vi "Write and Convert Waveform to File.vi"(0 "File Refnum":refnum<file>, 1 "Current Supplied Voltage":dbl, 2 "Calibration State":enum16{"Idle", "Delay", "Voltage", "Response"}(ring), 5 "Waveform":waveform(dbl)[](array[waveform]), 7 "Prev Array":dbl[][](array[numeric]), 11 "error in":errorcluster) -> (4 "File Refnum Out":refnum<file>, 6 "Bridge OP Out":dbl, 10 "Shunt Volt Out":dbl, 14 "Bridge & Volt array":dbl[][](array[numeric]), 15 "error out":errorcluster)   [LabVIEW 2021]
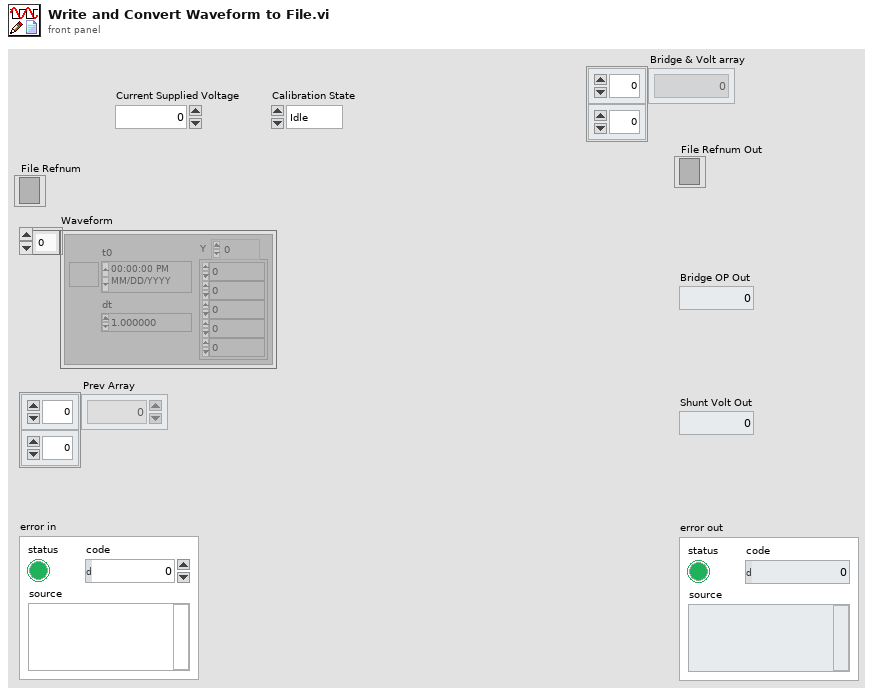
[diagram p1: front panel]
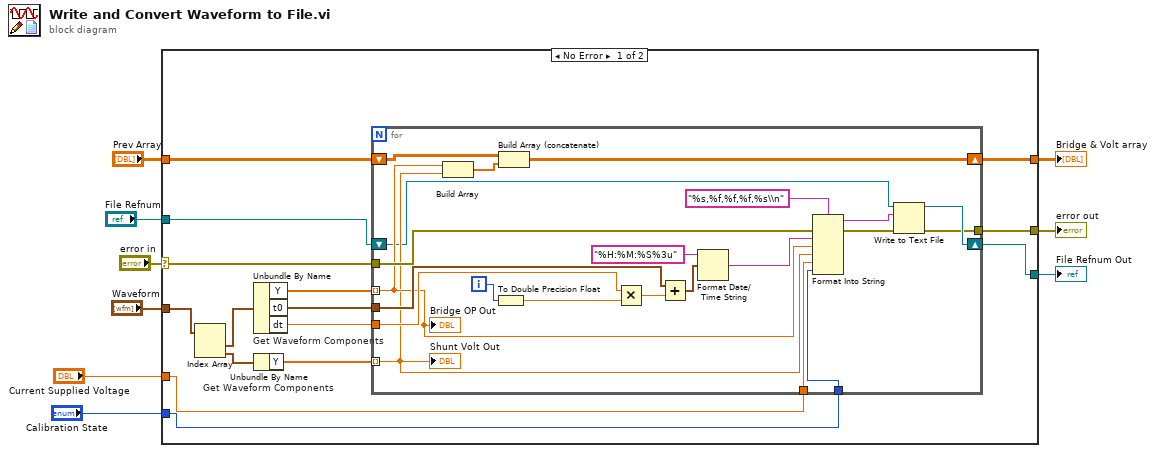
[diagram p0: block diagram]
diagram:
  n1 = case shown="No Error" "error in" {
    selector: "error in" -> [w24 w49]
    tunnel: "Waveform" -> [w14 _]
    tunnel: [w19 w49] -> w7
    tunnel: "File Refnum" -> [w23 w48]
    tunnel: [w22 w48] -> w5
    tunnel: "Prev Array" -> [w21 w47]
    tunnel: [w20 w47] -> w3
    tunnel: "Current Supplied Voltage" -> [w11 _]
    tunnel: "Calibration State" -> [w10 _]
    frame No Error {
      n2 = Index Array(array=w14) -> (element #1=w13:waveform(dbl), element #2=w12:waveform(dbl))  [unwired: 2 in]
      n3 = Unbundle By Name "Get Waveform Components"(w13) -> ("Y"=w18:dbl[], "t0"=w16:timestamp, "dt"=w17:dbl)
      n4 = Unbundle By Name "Get Waveform Components"(w12) -> ("Y"=w15:dbl[])
      n5 = for {
        tunnel: w18 -> [w31] mode=indexing
        tunnel: w17 -> [w44]
        tunnel: w24 -> [w42]
        shift-right: [w28] -> w22
        shift-left: w23 -> [w29]
        tunnel: w16 -> [w38]
        shift-right: [w33] -> w20
        shift-left: w21 -> [w34]
        tunnel: w15 -> [w30] mode=indexing
        tunnel: [w27] -> w19
        tunnel: w11 -> [w26]
        tunnel: w10 -> [w25]
        i -> [w46]
        n6 = Build Array(w31, w30) -> (w32:dbl[])
        n7 = To Double Precision Float(number=w46) -> (double precision float=w45:dbl)
        n8 = Build Array (concatenate)(w34, w32) -> (w33:dbl[][])
        n9 = Multiply(x=w44, y=w45) -> (x*y=w39:dbl)
        n10 = Add(x=w38, y=w39) -> (x+y=w37:timestamp)
        n11 = Format Date/Time String(time format string (%c)="%H:%M:%S%3u", seconds (now)=w37) -> (date/time string=w40:string)  [unwired: 1 in]
        n12 = Format Into String "Format Into String"(format string="%s,%f,%f,%f,%s\\n", error in=w42, w40, w31, w30, w26, w25) -> (resulting string=w35:string, error out=w36:errorcluster)  [unwired: 1 in]
        n13 = Write to Text File(file (use dialog)=w29, text=w35, error in=w36) -> (refnum out=w28:refnum<file>, error out=w27:errorcluster)  [unwired: 1 in, 1 out]
        "Bridge OP Out" <- w31
        "Shunt Volt Out" <- w30
      }
    }
    frame Error {
    }
  }
  "error out" <- w7
  "File Refnum Out" <- w5
  "Bridge & Volt array" <- w3
